vi "PathPlanner_Traectory_Test.vi"(8 "error in (no error)":errorcluster) -> (0 "error out":errorcluster, 3 "All Passed":bool)   [LabVIEW 2019]
uses:
  <vilib>/Rock Robotics/WPI/ThirdParty/JAS_Junk/TrajLib/Trajectory_Library.lvlib
  <vilib>/Rock Robotics/WPI/ThirdParty/MJansen/PathPlanner/PathPlanner24.lvlib
panel:
  out "Passed 1":bool
  # "Trajectory State"
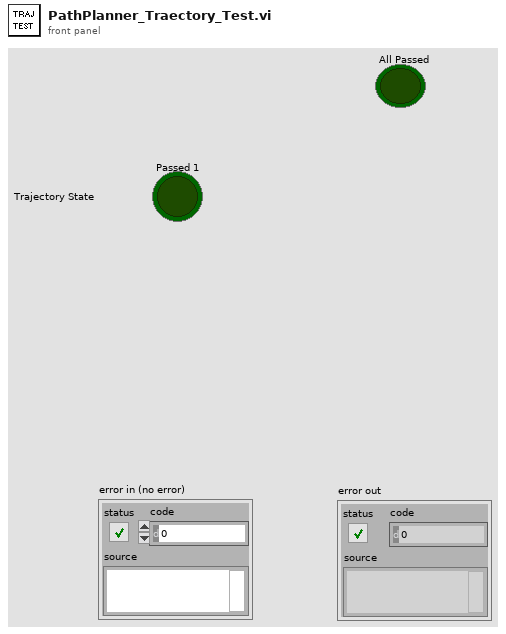
[diagram p1: front panel]
types:
  T1 = typedef "Trajectory_Library.lvlib/TRANSLATION2D.ctl" = cluster{"X":dbl, "Y":dbl}
  T2 = typedef "Trajectory_Library.lvlib/ROTATION2D.ctl" = cluster{"VALUE":dbl, "COS":dbl, "SIN":dbl}
  T3 = typedef "PathPlanner24.lvlib/PathPlannerPathConstraints.ctl" = cluster{"MaxVelocityMps;":dbl, "MaxAccelerationMpsSq;":dbl, "MaxAngularVelRadPsEc;":dbl, "MaxAngularAccRadPSecSq":dbl, "Exists":bool, "Unlimited":bool, "NominalVoltageVolts":dbl}
  T4 = typedef "PathPlanner24.lvlib/PathPlannerTrajectoryState.ctl" = cluster{"TimeSeconds":dbl, "VelocityMPS":dbl, "AccerationMpsSq":dbl, "HeadingAngularVelRadPerSec":dbl, "PositionMeters":T1, "Heading":T2, "TargetHolonomicRotation":T2, "CurvatureRadPerMeter":dbl, "PathPlannerConstraints":T3, "DeltaPos":dbl, "WaypointRelPos":dbl}
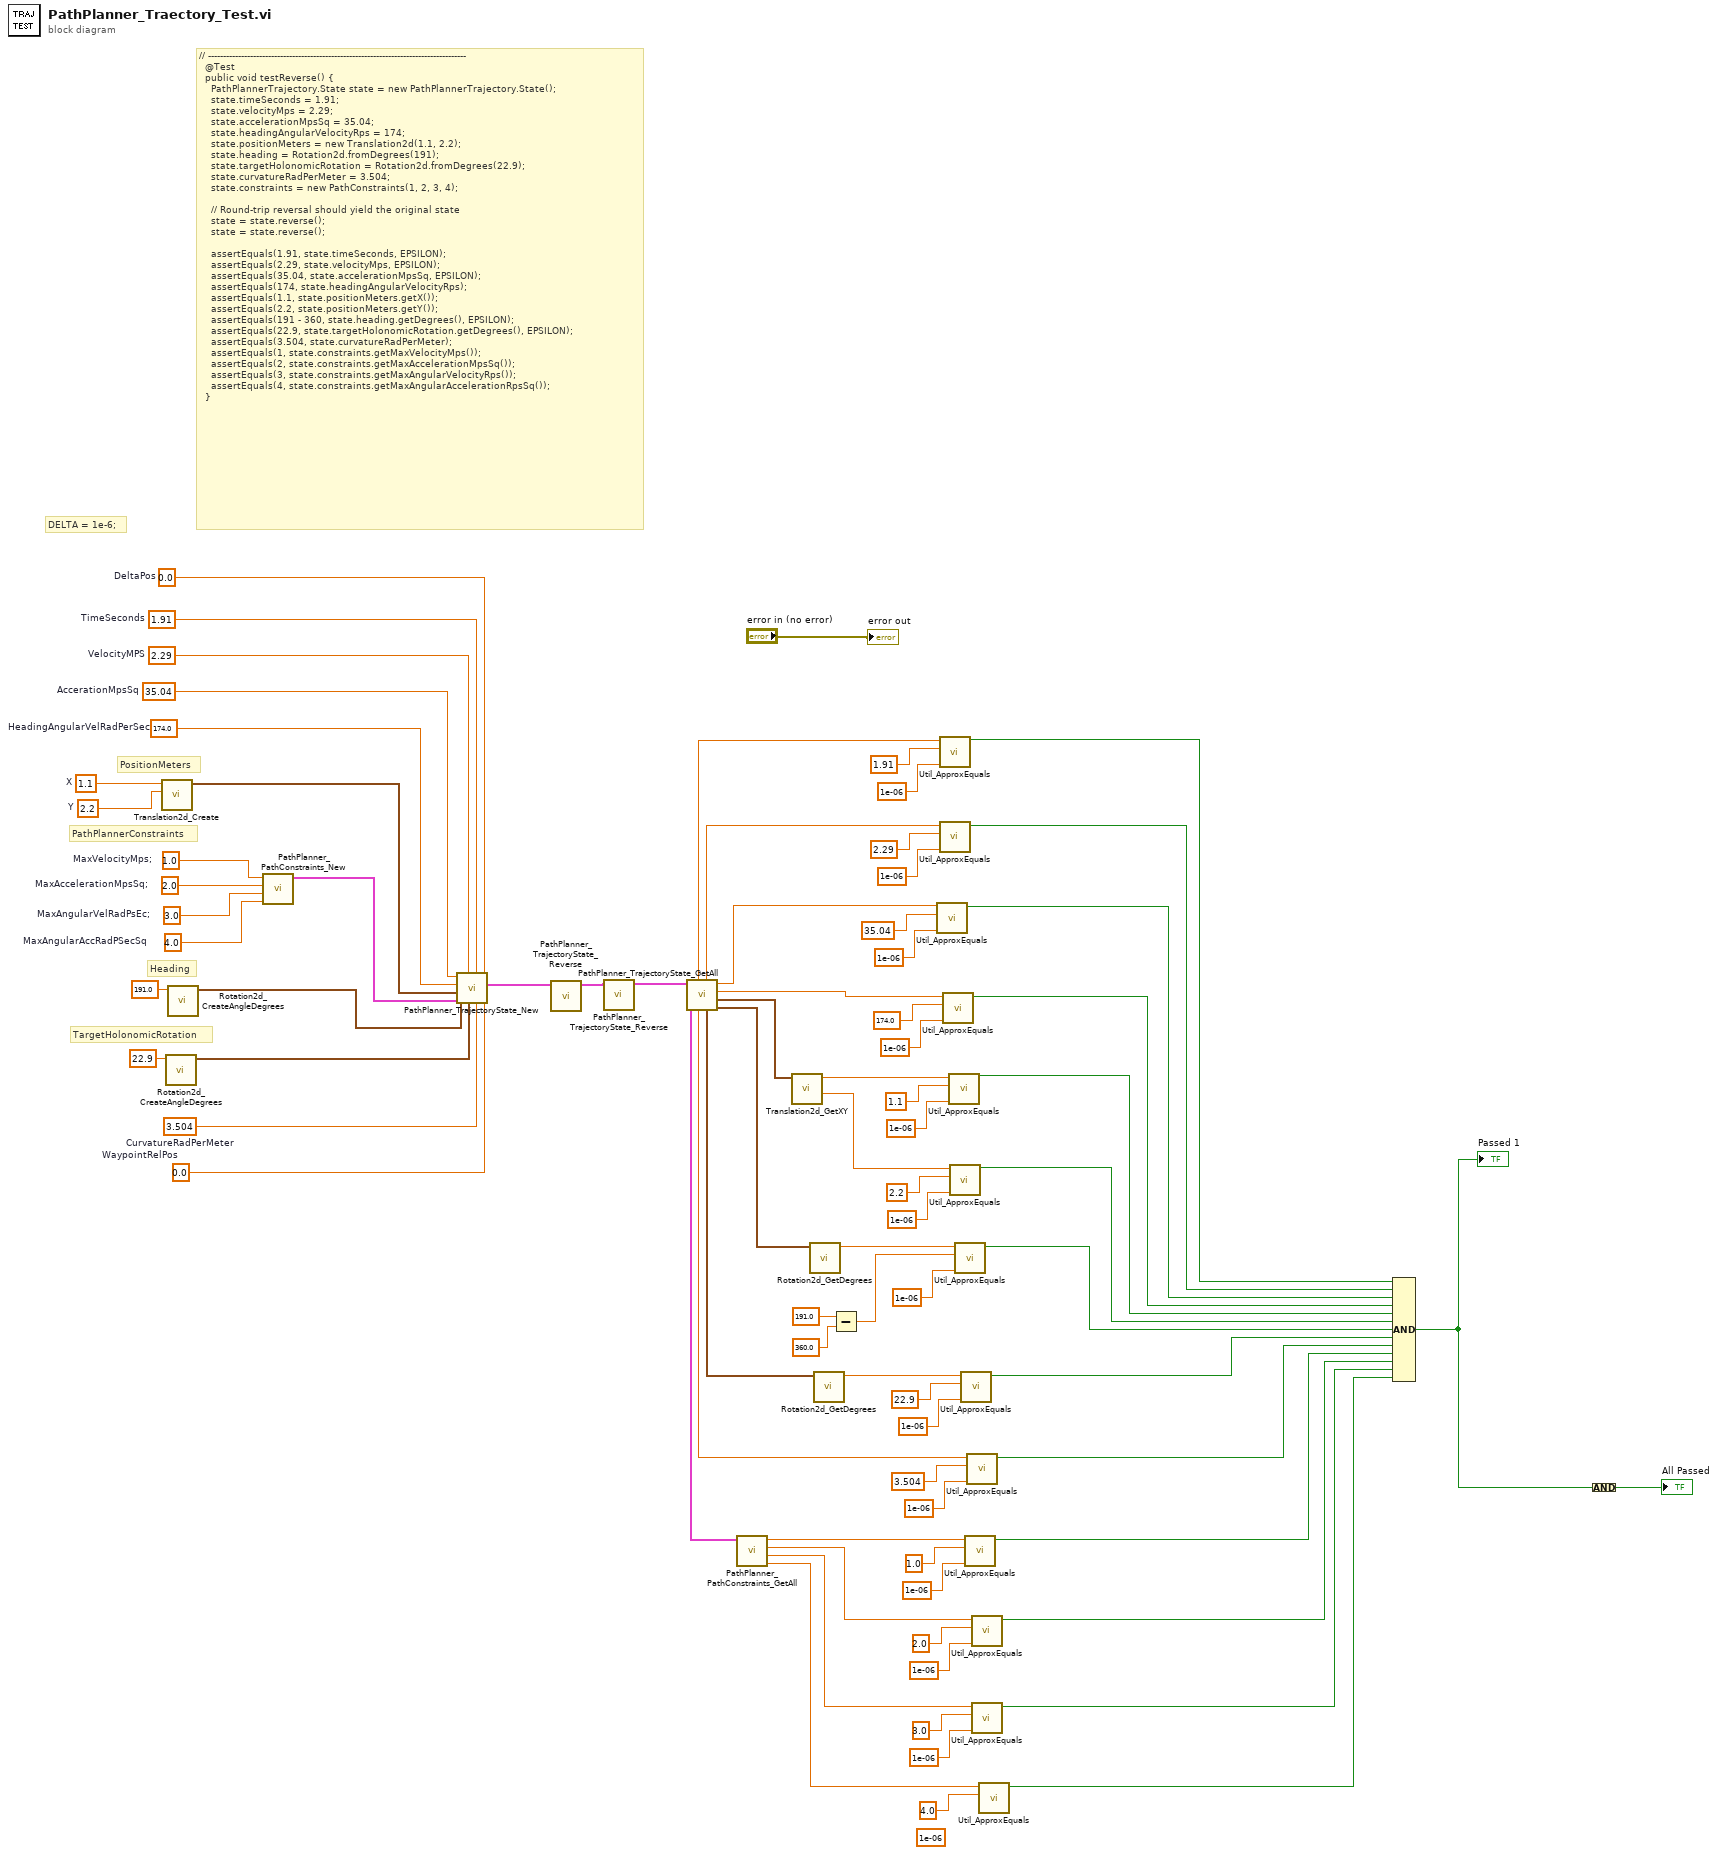
[diagram p0: block diagram]
diagram:
  w1 = 0.0  # WaypointRelPos
  (unwired) 1e-06 ("Tolerance")
  w51 = 1.0  # MaxVelocityMps;
  w52 = 2.0  # MaxAccelerationMpsSq;
  w53 = 3.0  # MaxAngularVelRadPsEc;
  w54 = 4.0  # MaxAngularAccRadPSecSq
  w57 = 1.1  # X
  w58 = 2.2  # Y
  w63 = 35.04  # AccerationMpsSq
  w64 = 174.0  # HeadingAngularVelRadPerSec
  w65 = 2.29  # VelocityMPS
  w66 = 1.91  # TimeSeconds
  w67 = 3.504  # CurvatureRadPerMeter
  w68 = 0.0  # DeltaPos
  # "PathPlannerConstraints"
  # "Heading"
  # "TargetHolonomicRotation"
  # "PositionMeters"
  # "// --------------------------------------------------------------------------------------\n  @Test\n  public void testReverse() {\n    PathPlannerTrajectory.State state = new PathPlannerTrajectory.State();\n    state.timeSeconds = 1.91;\n    state.velocityMps = 2.29;\n    state.accelerationMpsSq = 35.04;\n    state.headingAngularVelocityRps = 174;\n    state.positionMeters = new Translation2d(1.1, 2.2);\n    state.heading = Rotation2d.fromDegrees(191);\n    state.targetHolonomicRotation = Rotation2d.fromDegrees(22.9);\n    state.curvatureRadPerMeter = 3.504;\n    state.constraints = new PathConstraints(1, 2, 3, 4);\n\n    // Round-trip reversal should yield the original state\n    state = state.reverse();\n    state = state.reverse();\n\n    assertEquals(1.91, state.timeSeconds, EPSILON);\n    assertEquals(2.29, state.velocityMps, EPSILON);\n    assertEquals(35.04, state.accelerationMpsSq, EPSILON);\n    assertEquals(174, state.headingAngularVelocityRps);\n    assertEquals(1.1, state.positionMeters.getX());\n    assertEquals(2.2, state.positionMeters.getY());\n    assertEquals(191 - 360, state.heading.getDegrees(), EPSILON);\n    assertEquals(22.9, state.targetHolonomicRotation.getDegrees(), EPSILON);\n    assertEquals(3.504, state.curvatureRadPerMeter);\n    assertEquals(1, state.constraints.getMaxVelocityMps());\n    assertEquals(2, state.constraints.getMaxAccelerationMpsSq());\n    assertEquals(3, state.constraints.getMaxAngularVelocityRps());\n    assertEquals(4, state.constraints.getMaxAngularAccelerationRpsSq());\n  }"
  # "DELTA = 1e-6;"
  n1 = call <vilib>:"Translation2d_Create.vi"("Y"=w58, "X"=w57) -> ("TRANSLATION"=w62:T1)  [unwired: 9 in]
  n2 = call <vilib>:"Rotation2d_CreateAngleDegrees.vi"("Angle_Degrees"=22.9) -> ("ROTATION"=w59:T2)  [unwired: 10 in]
  n3 = call <vilib>:"Rotation2d_CreateAngleDegrees.vi"("Angle_Degrees"=191.0) -> ("ROTATION"=w60:T2)  [unwired: 10 in]
  n4 = call <vilib>:"PathPlanner_PathConstraints_New.vi"("MaxAngularAccRadPSecSq"=w54, "MaxAngularVelRadPsEc;"=w53, "MaxAccelerationMpsSq;"=w52, "MaxVelocityMps;"=w51) -> ("PathPlannerConstraints"=w61:T3)  [unwired: 7 in]
  n5 = call <vilib>:"PathPlanner_TrajectoryState_New.vi"("PathPlannerConstraints"=w61, "WaypointRelPos"=w1, "DeltaPos"=w68, "CurvatureRadPerMeter"=w67, "TimeSeconds"=w66, "TargetHolonomicRotation"=w59, "VelocityMPS"=w65, "Heading"=w60, "PositionMeters"=w62, "HeadingAngularVelRadPerSec"=w64, "AccerationMpsSq"=w63) -> ("PathPlannerState"=w69:T4)
  n6 = call <vilib>:"PathPlanner_TrajectoryState_Reverse.vi"("PathPlannerState"=w69) -> ("Reversed State"=w70:T4)  [unwired: 10 in]
  n7 = call <vilib>:"PathPlanner_TrajectoryState_Reverse.vi"("PathPlannerState"=w70) -> ("Reversed State"=w50:T4)  [unwired: 10 in]
  n8 = call <vilib>:"PathPlanner_TrajectoryState_GetAll.vi"("PathPlannerState"=w50) -> ("Heading"=w29:T2, "PositionMeters"=w34:T1, "HeadingAngularVelRadPerSec"=w35:dbl, "AccerationMpsSq"=w36:dbl, "TargetHolonomicRotation"=w24:T2, "VelocityMPS"=w39:dbl, "CurvatureRadPerMeter"=w20:dbl, "TimeSeconds"=w40:dbl, "PathPlannerConstraints"=w12:T3)  [unwired: 1 in, 1 out]
  n9 = call <vilib>:"PathPlanner_PathConstraints_GetAll.vi"("PathPlannerConstraints"=w12) -> ("MaxAngularAccRadPSecSq"=w13:dbl, "MaxAngularVelRadPsEc;"=w14:dbl, "MaxAccelerationMpsSq;"=w15:dbl, "MaxVelocityMps;"=w16:dbl)  [unwired: 6 in, 1 out]
  n10 = call <vilib>:"Translation2d_GetXY.vi"("In Translation"=w34) -> ("Y"=w30:dbl, "X"=w31:dbl)  [unwired: 9 in]
  n11 = call <vilib>:"Rotation2d_GetDegrees.vi"("in ROTATION"=w29) -> ("AngleDegrees"=w26:dbl)  [unwired: 10 in]
  n12 = call <vilib>:"Rotation2d_GetDegrees.vi"("in ROTATION"=w24) -> ("AngleDegrees"=w21:dbl)  [unwired: 10 in]
  n13 = Subtract(x=191.0, y=360.0) -> (x-y=w25:dbl)
  n14 = call <vilib>:"Util_ApproxEquals.vi"("Tolerance"=1e-06, "Value 2"=35.04, "Value 1"=w36) -> ("ApproxEquals"=w6:bool)  [unwired: 8 in]
  n15 = call <vilib>:"Util_ApproxEquals.vi"("Tolerance"=1e-06, "Value 2"=1.91, "Value 1"=w40) -> ("ApproxEquals"=w4:bool)  [unwired: 8 in]
  n16 = call <vilib>:"Util_ApproxEquals.vi"("Tolerance"=1e-06, "Value 2"=2.29, "Value 1"=w39) -> ("ApproxEquals"=w5:bool)  [unwired: 8 in]
  n17 = call <vilib>:"Util_ApproxEquals.vi"("Tolerance"=1e-06, "Value 2"=174.0, "Value 1"=w35) -> ("ApproxEquals"=w7:bool)  [unwired: 8 in]
  n18 = call <vilib>:"Util_ApproxEquals.vi"("Tolerance"=1e-06, "Value 2"=1.1, "Value 1"=w31) -> ("ApproxEquals"=w8:bool)  [unwired: 8 in]
  n19 = call <vilib>:"Util_ApproxEquals.vi"("Tolerance"=1e-06, "Value 2"=2.2, "Value 1"=w30) -> ("ApproxEquals"=w9:bool)  [unwired: 8 in]
  n20 = call <vilib>:"Util_ApproxEquals.vi"("Tolerance"=1e-06, "Value 2"=w25, "Value 1"=w26) -> ("ApproxEquals"=w10:bool)  [unwired: 8 in]
  n21 = call <vilib>:"Util_ApproxEquals.vi"("Tolerance"=1e-06, "Value 2"=22.9, "Value 1"=w21) -> ("ApproxEquals"=w11:bool)  [unwired: 8 in]
  n22 = call <vilib>:"Util_ApproxEquals.vi"("Tolerance"=1e-06, "Value 2"=1.0, "Value 1"=w16) -> ("ApproxEquals"=w74:bool)  [unwired: 8 in]
  n23 = call <vilib>:"Util_ApproxEquals.vi"("Tolerance"=1e-06, "Value 2"=3.504, "Value 1"=w20) -> ("ApproxEquals"=w80:bool)  [unwired: 8 in]
  n24 = call <vilib>:"Util_ApproxEquals.vi"("Tolerance"=1e-06, "Value 2"=2.0, "Value 1"=w15) -> ("ApproxEquals"=w71:bool)  [unwired: 8 in]
  n25 = call <vilib>:"Util_ApproxEquals.vi"("Tolerance"=1e-06, "Value 2"=3.0, "Value 1"=w14) -> ("ApproxEquals"=w3:bool)  [unwired: 8 in]
  n26 = call <vilib>:"Util_ApproxEquals.vi"("Value 2"=4.0, "Value 1"=w13) -> ("ApproxEquals"=w2:bool)  [unwired: 9 in]
  n27 = Compound Arithmetic op=AND(w4, w5, w6, w7, w8, w9, w10, w11, w80, w74, w71, w3, w2) -> (w79:bool)
  "Passed 1" <- w79
  n28 = Compound Arithmetic op=AND(w79) -> (→"All Passed":bool)
  "error out" <- "error in (no error)"
